vi "forceToVoltage.vi"(8 "error in (no error)":errorcluster, 10 "Force":dbl[unit], 11 "ForceToFlowControlVoltage in":refnum<class "ForceToFlowControlVoltage.lvclass">) -> (0 "error out":errorcluster, 2 "Voltage":dbl[unit], 3 "ForceToFlowControlVoltage out":refnum<class "ForceToFlowControlVoltage.lvclass">)   [LabVIEW 2015, in "ForceToFlowControlVoltage.lvclass"]
uses:
  ForceToFlowControlVoltage.lvclass
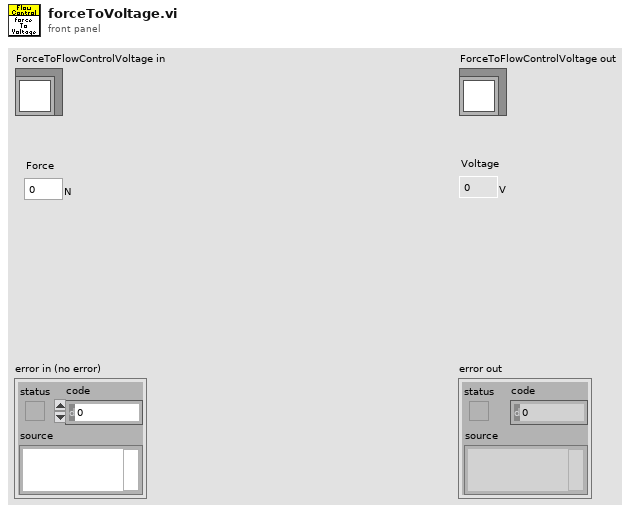
[diagram p1: front panel]
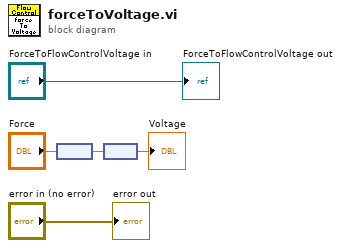
[diagram p0: block diagram]
diagram:
  n1 = node("Force") -> (w2:dbl)
  n2 = node(w2) -> (→"Voltage":dbl[unit])
  "error out" <- "error in (no error)"
  "ForceToFlowControlVoltage out" <- "ForceToFlowControlVoltage in"
